vi "Image FT_find peak (SubVI).vi"(8 "error in (no error)":errorcluster, 10 "Array":sgl[](array[numeric]), 11 "Refnum in":T1) -> (0 "error out":errorcluster, 1 "Amplitudes":dbl[](array[numeric]) format="%.2p", 2 "Locations":dbl[](array[numeric]) format="%.2p", 3 "Power Spectrum":dbl[](array[numeric]), 5 "Pixels Line (U8)":u8[](array[numeric]), 6 "# found":i32, 7 "Waveform Graph 2":dbl[](graph))   [LabVIEW 2014]
uses:
  <vilib>/vision/Image Controls.llb/IMAQ Image.ctl
  <vilib>/Analysis/2dsp.llb/Power Spectrum (DBL).vi
  <vilib>/measure/mamon.llb/Waveform Peak Detection for 1 Chan.vi
  <vilib>/Analysis/NI_AALPro.lvlib
  <vilib>/measure/NI_MAPro.lvlib
  <vilib>/vision/NI_Vision_Development_Module.lvlib
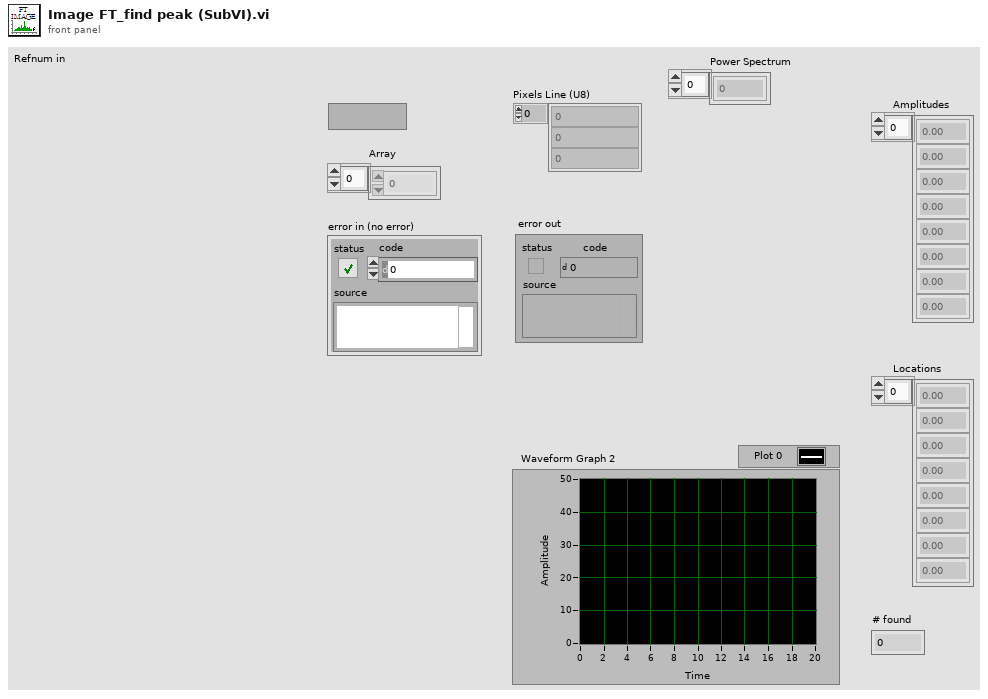
[diagram p1: front panel]
types:
  T1 = typedef "IMAQ Image.ctl" = refnum<image>
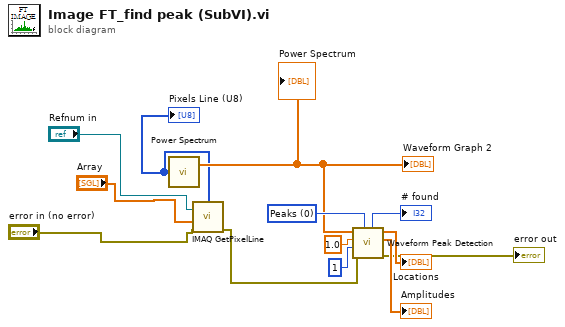
[diagram p0: block diagram]
diagram:
  w13 = u16 0 items=["Peaks", "Valleys"] ("peaks/valleys")
  n1 = call "IMAQ GetPixelLine"("error in (no error)"="error in (no error)", "Line Coordinates"="Array", "Image"="Refnum in") -> ("error out"=w2:errorcluster, "Pixels Line (U8)"=w3:u8[])  [unwired: 1 in, 3 out]
  "Pixels Line (U8)" <- w3
  n2 = call-poly <vilib>:"Power Spectrum.vi"("X"=w3) -> ("Power Spectrum"=w10:dbl[])  [unwired: 1 out]
  "Waveform Graph 2" <- w10
  "Power Spectrum" <- w10
  n3 = call-poly <vilib>:"Waveform Peak Detection.vi"("peaks/valleys"=w13, "error in"=w2, "width"=1, "threshold"=1.0, "Signal In"=w10) -> ("error out"=→"error out":errorcluster, "Amplitudes"=→"Amplitudes":dbl[], "Locations"=→"Locations":dbl[], "# found"=→"# found":i32)  [unwired: 2 in, 1 out]
